vi "FdxCmdTxQueueWriteExCvi.vi"(8 "error in":errorcluster, 9 "FrameEDE":T2 {"FrameType" items=["FDX_TX_FRAME_STD", "FDX_TX_FRAME_INSTR"]; "SequenceNumberOffset" items=["FDX_TX_FRAME_SEQ_OFFS_AUTO "=65535]; "SequenceNumberInit" items=["FDX_TX_FRAME_SEQ_INIT_AUTO"=65535]; "PhysErrorInjection" items=["FDX_TX_FRAME_ERR_OFF"=0, "FDX_TX_FRAME_ERR_CRC"=1, "FDX_TX_FRAME_ERR_ALI"=2, "FDX_TX_FRAME_ERR_PRE"=4, "FDX_TX_FRAME_ERR_PHY"=8]; "FrameStartMode" items=["FDX_TX_FRAME_START_IFG", "FDX_TX_FRAME_START_PGWT", "FDX_TX_FRAME_START_TRG"]; "NetSelect" items=["FDX_TX_FRAME_DLY_A"=0, "FDX_TX_FRAME_DLY_B"=1, "FDX_TX_FRAME_BOTH "=3, "FDX_TX_FRAME_ONLY_A"=4, "FDX_TX_FRAME_ONLY_B "=5]; "PreambleCount" max=15; "ExternalStrobe" items=["FDX_DIS", "FDX_ENA"]; "PayloadGenerationMode" items=["FDX_TX_FRAME_PGM_USER"=0, "FDX_TX_FRAME_PGM_IP_PART"=1, "FDX_TX_FRAME_PGM_IP_FULL"=2, "FDX_TX_FRAME_PGM_IP_PART_TT"=10, "FDX_TX_FRAME_PGM_IP_FULL_TT"=20]; "PayloadBufferMode" items=["FDX_TX_FRAME_PBM_STD", "FDX_TX_FRAME_PBM_MAC", "FDX_TX_FRAME_PBM_UDP"]}, 10 "FrameHeaderEDE":T1 {"HeaderType" items=["FDX_TX_FRAME_HEADER_GENERIC ", "FDX_TX_FRAME_HEADER_REPLAY"]}, 11 "InstrumentHandle":u32) -> (0 "error out":errorcluster, 3 "InstrumentHandle":u32)   [LabVIEW 2020, in "AIM664LV.lvlib"]
doc: "This function is used to write Entries to a Transmit Queue from a provided buffer. For this write function the number of Entries and the number of bytes to write needs to be specified. The entries will always be queued at the end of the transmit queue."
uses:
  AIM664LV.lvlib
  AFDX_LibraryAdmin/FdxGlobalDllPath.vi
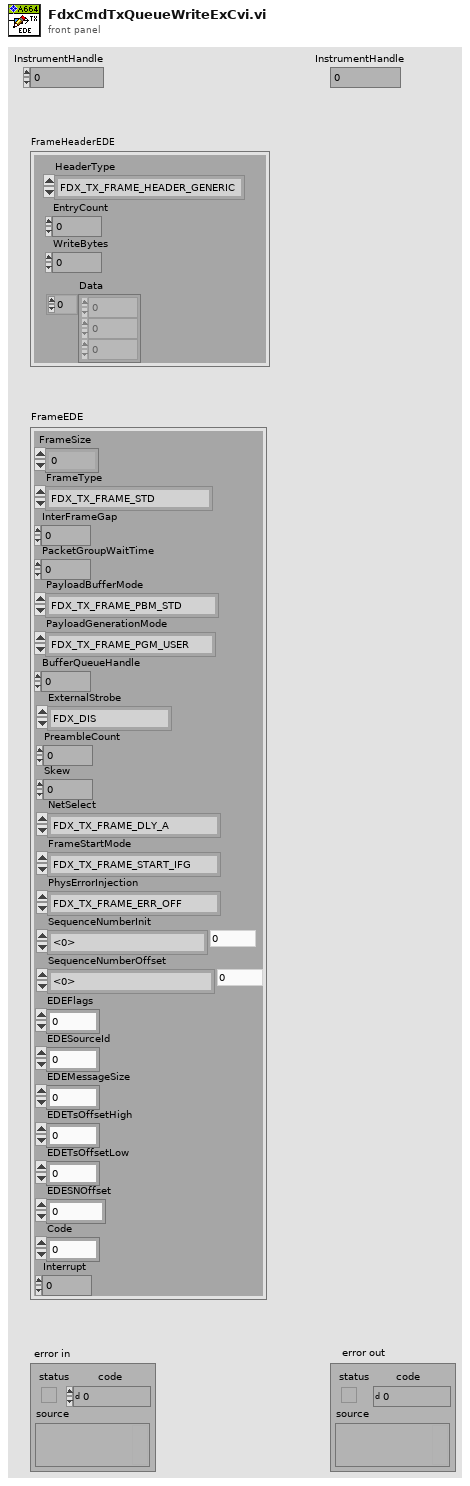
[diagram p1: front panel]
types:
  T1 = cluster{"HeaderType":u32, "EntryCount":u32, "WriteBytes":u32, "Data":u8[]}
  T2 = cluster{"FrameSize":u16, "FrameType":u8, "InterFrameGap":u32, "PacketGroupWaitTime":u32, "PayloadBufferMode":u8, "PayloadGenerationMode":u8, "BufferQueueHandle":u32, "ExternalStrobe":u8, "PreambleCount":u8, "Skew":u32, "NetSelect":u8, "FrameStartMode":u8, "PhysErrorInjection":u32, "SequenceNumberInit":u16, "SequenceNumberOffset":u16, "EDEFlags":u32, "EDESourceId":u32, "EDEMessageSize":u32, "EDETsOffsetHigh":u32, "EDETsOffsetLow":u32, "EDESNOffset":u32, "Code":u8, "Interrupt":u8}
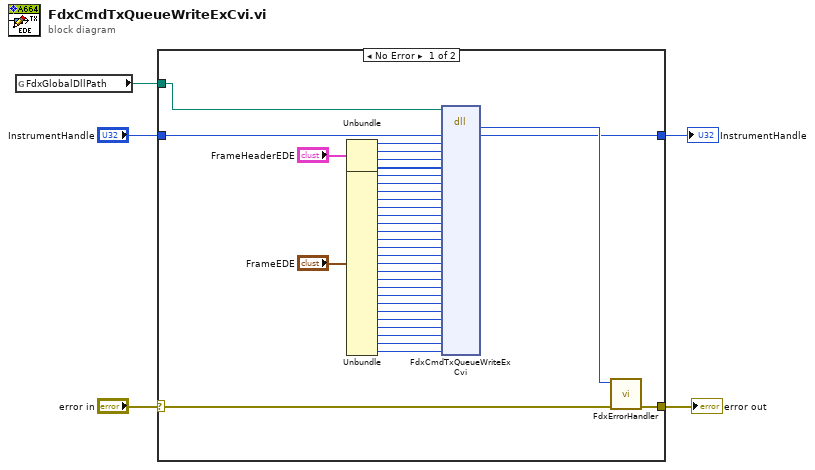
[diagram p0: block diagram]
diagram:
  n1 = global read "FdxGlobalDllPath.vi" "FdxGlobalDllPath"() -> (w3:path)
  n2 = case shown="No Error" "error in" {
    selector: "error in" -> [w39 w42]
    tunnel: [w40 w42] -> w5
    tunnel: w3 -> [w8 _]
    tunnel: [w7 w41] -> w2
    tunnel: "InstrumentHandle" -> [w6 w41]
    frame No Error {
      n3 = Unbundle("FrameHeaderEDE") -> ("HeaderType"=w24:u32, "EntryCount"=w23:u32, "WriteBytes"=w22:u32, "Data"=w21:u8[])
      n4 = Unbundle("FrameEDE") -> ("FrameSize"=w36:u16, "FrameType"=w35:u8, "InterFrameGap"=w34:u32, "PacketGroupWaitTime"=w33:u32, "PayloadBufferMode"=w26:u8, "PayloadGenerationMode"=w32:u8, "BufferQueueHandle"=w31:u32, "ExternalStrobe"=w30:u8, "PreambleCount"=w29:u8, "Skew"=w28:u32, "NetSelect"=w27:u8, "FrameStartMode"=w20:u8, "PhysErrorInjection"=w19:u32, "SequenceNumberInit"=w18:u16, "SequenceNumberOffset"=w17:u16, "EDEFlags"=w16:u32, "EDESourceId"=w15:u32, "EDEMessageSize"=w14:u32, "EDETsOffsetHigh"=w13:u32, "EDETsOffsetLow"=w12:u32, "EDESNOffset"=w11:u32, "Code"=w10:u8, "Interrupt"=w9:u8)
      n5 = dll-call lib="aim_fdx.19.dll" fn="FdxCmdTxQueueWriteExCvi"(path in=w8, "InstrumentHandle"=w6, "HeaderType"=w24, "EntryCount"=w23, "WriteBytes"=w22, "Data"=w21, "FrameSize"=w36, "FrameType"=w35, "InterFrameGap"=w34, "PacketGroupWaitTime"=w33, "PayloadBufferMode"=w26, "PayloadGenerationMode"=w32, "BufferQueue Handle"=w31, "ExternalStrobe"=w30, "PreambleCount"=w29, "Skew"=w28, "NetSelect"=w27, "FrameStartMode"=w20, "PhysErrorInjection"=w19, "SequenceNumberInit"=w18, "SequenceNumberOffset"=w17, "EDEFlags"=w16, "EDESourceId"=w15, "EDEMessageSize"=w14, "EDETsOffsetHigh"=w13, "EDETsOffsetLow"=w12, "EDESNOffset"=w11, "Code"=w10, "Interrupt"=w9) -> ("status"=w38:i32, "InstrumentHandle"=w7:u32)  [unwired: 29 in, 2 out]
      n6 = call "FdxErrorHandler.vi"("error in"=w39, "AIM Error"=w38) -> ("error out"=w40:errorcluster)  [unwired: 9 in]
    }
    frame Error {
    }
  }
  "error out" <- w5
  "InstrumentHandle" <- w2
